vi "Serial_Write.vi"(8 "error in (no error)":errorcluster, 9 "Text to write":string, 11 "Python":T1) -> (0 "error out":errorcluster)   [LabVIEW 2020]
uses:
  PythonCtrl.ctl
panel:
  out "result string":string
  out "Num loops":i32
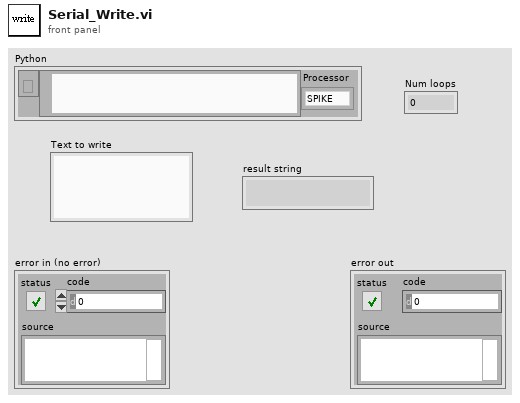
[diagram p1: front panel]
types:
  T1 = typedef "PythonCtrl.ctl" = cluster{"session":refnum<k35>, "PyPath":path, "Processor":enum16{"SPIKE", "Pi"}}
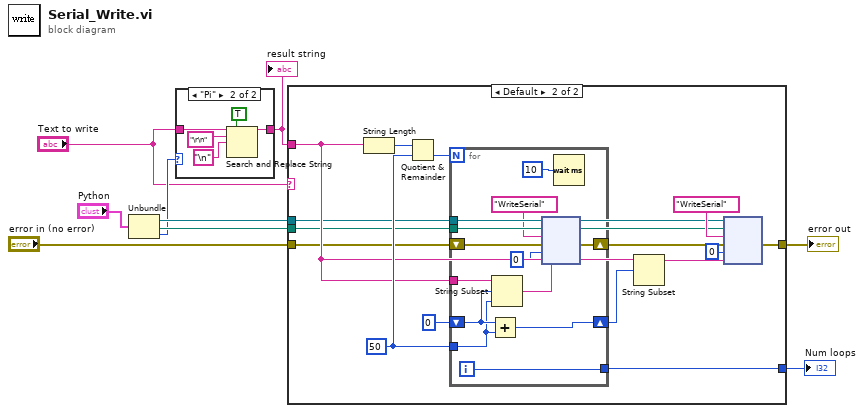
[diagram p0: block diagram]
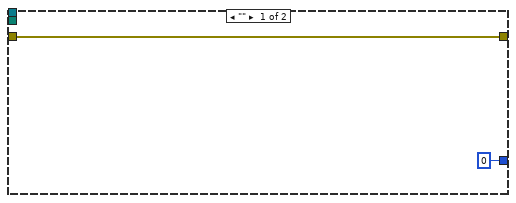
[diagram p3: hidden frame]
diagram:
  n1 = Unbundle("Python") -> ("session"=w5:refnum<k35>, "PyPath"=w4:path, "Processor"=w3:enum16{"SPIKE", "Pi"})
  n2 = case shown="\"Pi\"" w3 {
    tunnel: "Text to write" -> [w10 w15]
    tunnel: [w10 w14] -> w1
    frame "SPIKE", Default {
    }
    frame "Pi" {
      n3 = Search and Replace String(replace all?=TRUE ("replace all? (F)"), input string=w15, search string="\r\n" ("regular expression"), replace string="\n" ("regular expression")) -> (result string=w14:string)  [unwired: 4 in, 3 out]
    }
  }
  "result string" <- w1
  n4 = case shown="Default" "Text to write" {
    tunnel: [0 w27] -> w9
    tunnel: w1 -> [_ w26]
    tunnel: "error in (no error)" -> [w17 w25]
    tunnel: [w17 w20] -> w7
    tunnel: w5 -> [_ w19]
    tunnel: w4 -> [_ w18]
    frame "" {
    }
    frame Default {
      w30 = 50 ("length (rest)")
      n5 = String Length(string=w26) -> (length=w29:i32)
      n6 = Quotient & Remainder(x=w29, y=w30) -> (floor(x/y)=w31:i32)  [unwired: 1 out]
      n7 = for {
        N: w31 -> [_]
        tunnel: w26 -> [w45]
        shift-right: [w43] -> w32
        shift-left: 0 -> [w44]
        tunnel: w30 -> [w42]
        tunnel: [w40] -> w27
        shift-right: [w37] -> w22
        shift-left: w25 -> [w36]
        tunnel: w19 -> [w34]
        tunnel: w18 -> [w33]
        i -> [w40]
        n8 = Add(x=w44, y=w42) -> (x+y=w43:i32)
        n9 = String Subset(string=w45, offset (0)=w44, length (rest)=w42) -> (substring=w38:string)
        n10 = node(w34, w33, "WriteSerial" ("function name"), w36, 0, w38) -> (w37:errorcluster)  [unwired: 2 in, 3 out]
        n11 = Wait (ms)(milliseconds to wait=u32 10) -> ()  [unwired: 1 out]
      }
      n12 = String Subset(string=w26, offset (0)=w32) -> (substring=w21:string)  [unwired: 1 in]
      n13 = node(w19, w18, "WriteSerial" ("function name"), w22, 0, w21) -> (w20:errorcluster)  [unwired: 2 in, 3 out]
    }
  }
  "error out" <- w7
  "Num loops" <- w9
